vi "Grabber.vi"() -> ()   [LabVIEW 2013]
uses:
  <vilib>/userdefined/High Color/IMAQdx.ctl
  <vilib>/vision/Image Controls.llb/IMAQ Image.ctl
  CameraLan.lvclass
  <instrlib>/niHWS/nihws.llb/niHWS Open File Permissions ID.ctl
  <vilib>/Analysis/baseanly.llb/Mean (DBL).vi
  <vilib>/DAQmx/write.llb/DAQmx Write (Digital Bool 1Line 1Point).vi
  <vilib>/DAQmx/read.llb/DAQmx Read (Digital Bool 1Line 1Point).vi
  <instrlib>/niHWS/nihws.llb/niHWS Write Analog WDT.vi
  <instrlib>/niHWS/nihws.llb/niHWS Write Analog DBL.vi
  <vilib>/DAQmx/miscellaneous.llb/DAQmx Fill In Error Info.vi
  <vilib>/vision/NI_Vision_Development_Module.lvlib
  <vilib>/Analysis/NI_AALBase.lvlib
  <vilib>/ptbypt/NI_PtbyPt.lvlib
panel:
  out "ElectricalTrace 2":dbl format="%0.2f"
  in  "Threshold":dbl=4.0 format="%#_13g"
  in  "Sample":bool
  in  "Method":u16(ring) items=["Electrical/Optical"=3, "Electrical"=2, "Optical"=1, "Electrical+Optical"=0]
  out "Lick":bool
  out "Resistance \n      Lick":bool
  out "mean":dbl format="%0.2f"
  out "std":dbl format="%0.2f"
  out "ElectricalTrace":dynamicdata(graph)
  in  "Threshold":dbl=0.8 format="%#_13g"
  out "Crop Error":errorcluster
  out "Crop":T1(plugin-control)
  out "OpticalTrace":dbl(graph)
  out "Camera\n    Lick":bool
  in  "Lick \nDetection":bool
  in  "Display":bool
  out "Image Out":T1
  in  "Default path":string="F:\\Camera\\"
  out "Juice":bool
  in  "ExposureTime":dbl(slide)=1000.0 caption="Gain" scale=0.0..16466.666666666668
  in  "Magnify":bool
  in  "stop":bool
  in  "Compressor":string(combo)="DV Video Encoder"
  in  "quality":i32=-1
  in  "Rec":bool
  in  "Path":path
  in  "Gain":dbl(slide)=2.9811320754716983 min=1.0 max=16466.666666666668 scale=1.0..4.0
  out "acquired FPS":dbl
  out "Image":T1(plugin-control)
  in  "Session In":T2="S1028197"
  in  "Fps":i32=60
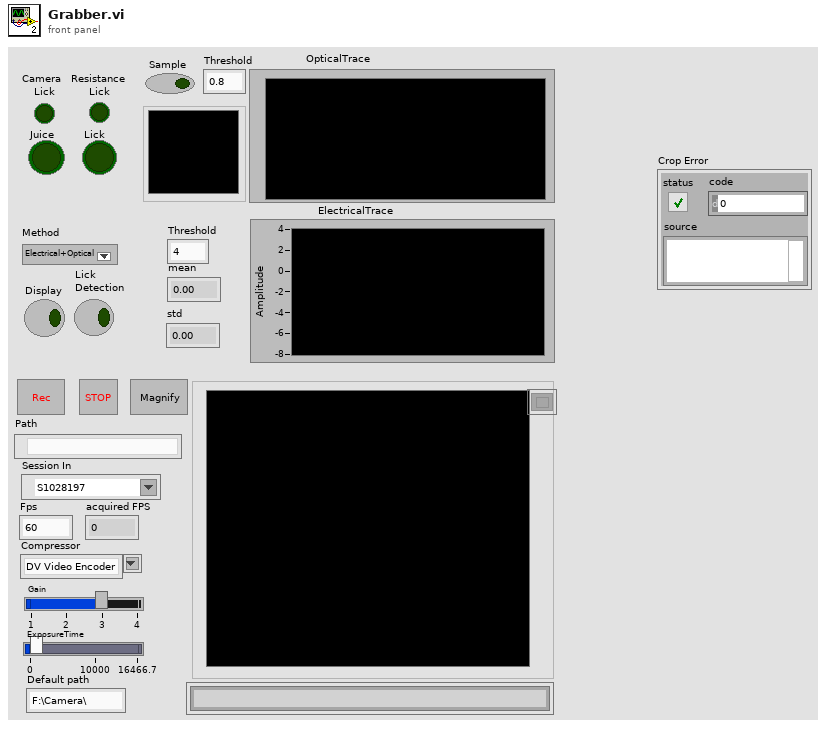
[diagram p1: front panel]
types:
  T1 = typedef "IMAQ Image.ctl" = refnum<image>
  T2 = typedef "IMAQdx.ctl" = refnum<k21>
  T3 = enum32{"Invalid", "Standard", "Closed", "Hidden", "Minimized", "Maximized"}
  T4 = typedef "niHWS Open File Permissions ID.ctl" = enum32{"Read Only", "Read/Write Existing", "Read/Write/Create New", "Read/Write/Create New Always"}
  T5 = typedef "AviRefnum.ctl" = refnum<k1>
  T6 = cluster{"Global Rectangle":i32[], "Contours":cluster{"Contour Type":u32, "ROI Type":u32, "Points":i32[]}[]}
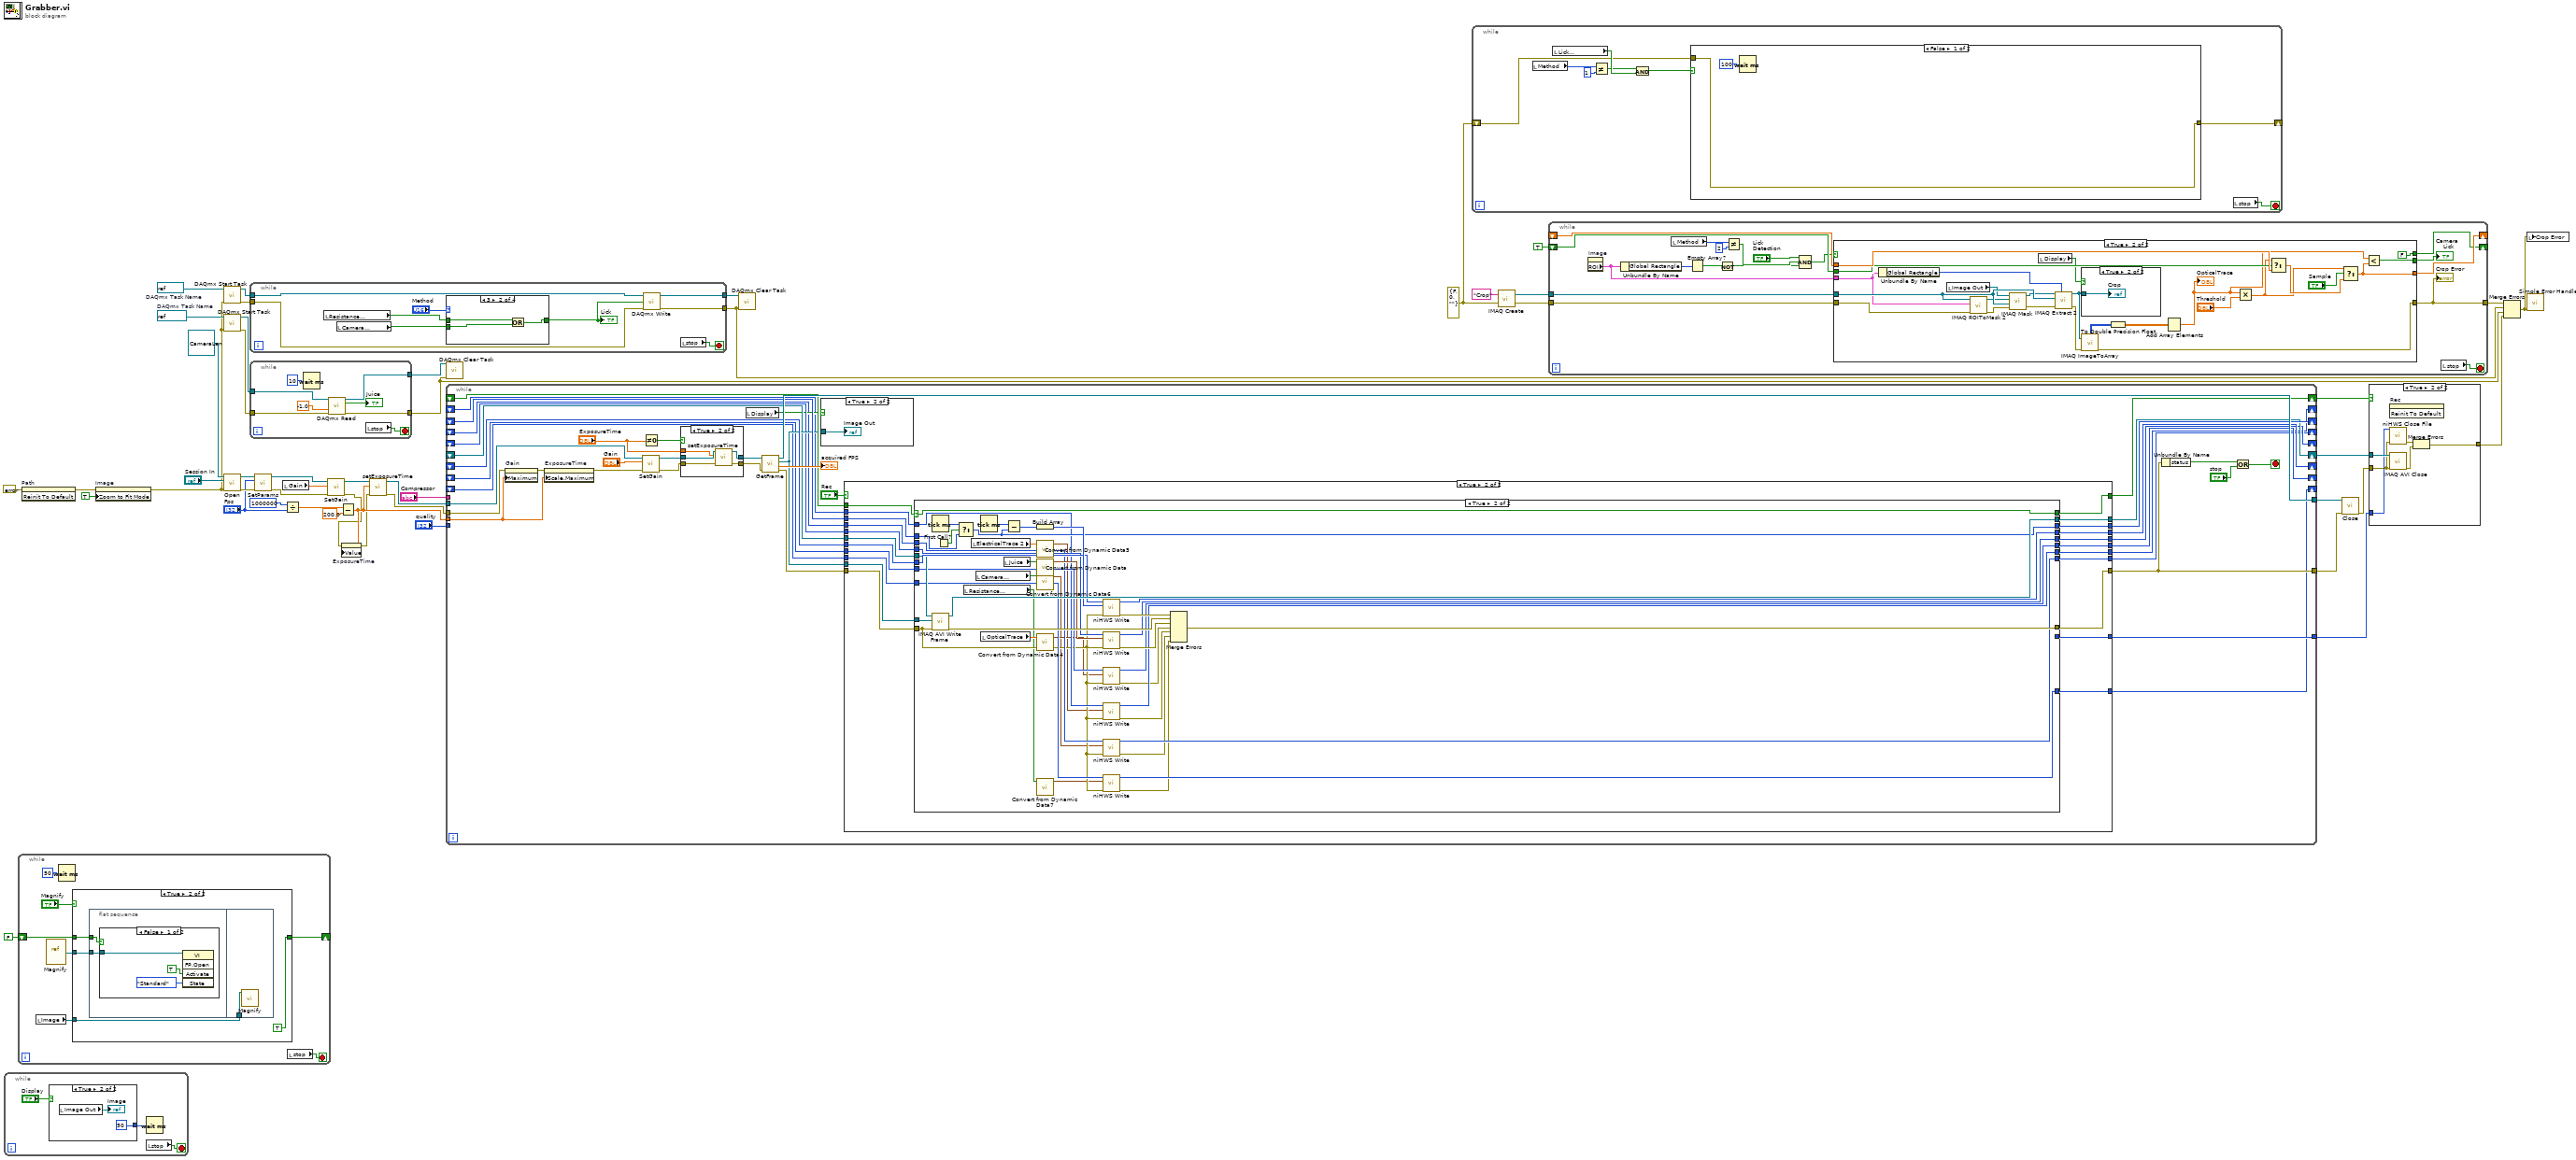
[diagram p0: block diagram]
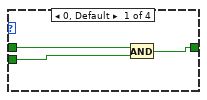
[diagram p2: hidden frame]
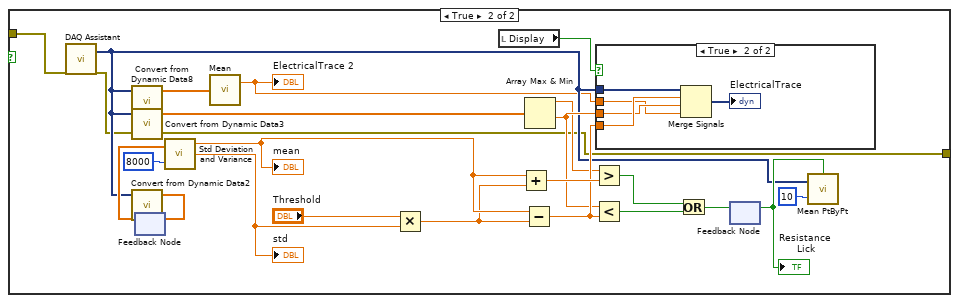
[diagram p5: hidden frame]
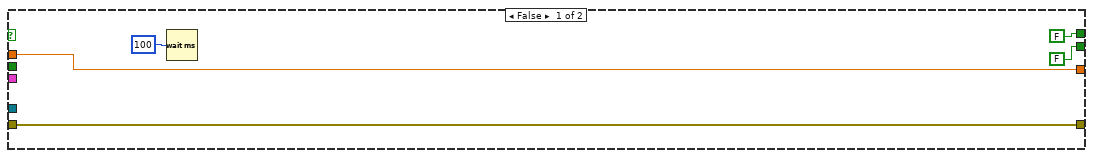
[diagram p7: hidden frame]
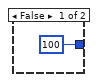
[diagram p9: hidden frame]
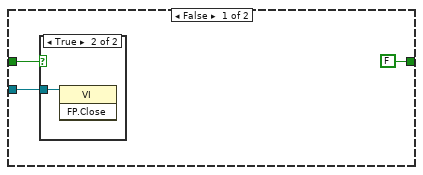
[diagram p10: hidden frame]
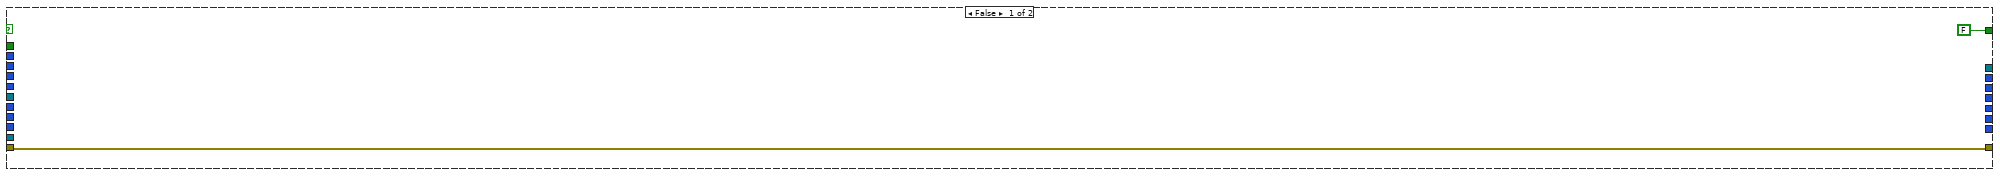
[diagram p16: hidden frame]
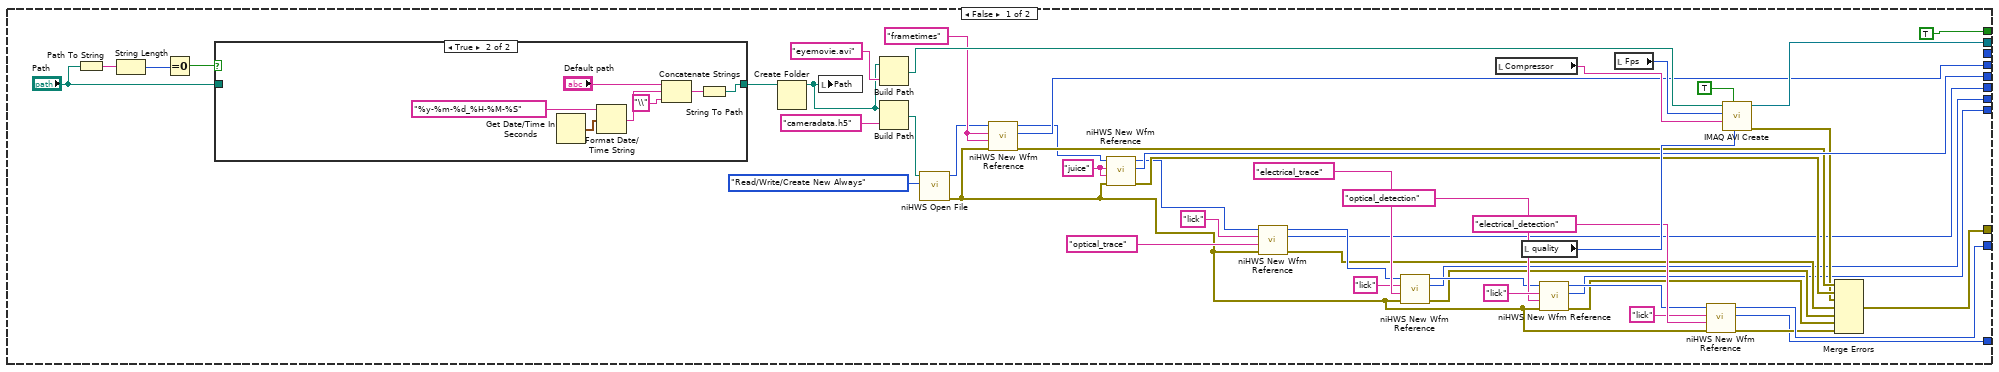
[diagram p17: hidden frame]
diagram:
  w21 = refnum<k21> "Lick"  # DAQmx Task Name
  w15 = errorcluster {"status"=FALSE, "code"=0, "source"=""} ("error in (no error)")
  w32 = refnum<k21> "Juice"  # DAQmx Task Name
  n1 = while {
    stop <- w51 stop-if-true
    n2 = case shown="True" "Display" {
      tunnel: [u32 100 ("milliseconds to wait") u32 50 ("milliseconds to wait")] -> w50
      frame False {
      }
      frame True {
        n3 = local read "Image Out"() -> (→"Image":T1)
      }
    }
    n4 = Wait (ms)(milliseconds to wait=w50) -> ()  [unwired: 1 out]
    n5 = local read "stop"() -> (w51:bool)
  }
  n6 = while {
    shift-right: [w59] -> _
    shift-left: FALSE -> [w58]
    stop <- w56 stop-if-true
    n7 = local read "Image"() -> (w55:T1)
    n8 = vi-ref "Magnify.vi"() -> (w61:refnum<vi>)
    n9 = Wait (ms)(milliseconds to wait=u32 50) -> ()  [unwired: 1 out]
    n10 = case shown="True" "Magnify" {
      tunnel: w61 -> [w64 w69]
      tunnel: [FALSE TRUE] -> w59
      tunnel: w58 -> [w63 w67]
      tunnel: w55 -> [_ w66]
      frame False {
        n11 = case shown="True" w63 {
          tunnel: w64 -> [_ w65]
          frame False {
          }
          frame True {
            n12 = invoke class="VI" method="FP.Close"(reference=w65) -> ()  [unwired: 2 in, 3 out]
          }
        }
      }
      frame True {
        n13 = flat-sequence {
          tunnel: w69 -> [w71]
          tunnel: w67 -> [w70]
          tunnel: w66 -> [w75]
          frame #0 {
            n14 = case shown="False" w70 {
              tunnel: w71 -> [w73 _]
              frame False {
                n15 = invoke class="VI" method="FP.Open"(reference=w73, "Activate"=TRUE ("Wait Until Done"), "State"=T3."Standard") -> ()  [unwired: 2 in, 5 out]
              }
              frame True {
              }
            }
          }
          frame #1 {
            n16 = call "Magnify.vi"("Camera 2"=w75) -> ()  [unwired: 11 in]
          }
        }
      }
    }
    n17 = local read "stop"() -> (w56:bool)
  }
  n18 = invoke on="Path" class="Path" method="Reinit To Default"(error in=errorcluster {"status"=FALSE, "code"=0, "source"=""} ("error in (no error)")) -> (error out=w22:errorcluster)  [unwired: 2 in, 2 out]
  n19 = property on="Image" class="ImageControl"(error in=w22, "Zoom to Fit Mode"=TRUE) -> (error out=w17:errorcluster)  [unwired: 1 in, 1 out]
  n20 = call <vilib>:"DAQmx Start Task.vi"("task/channels in"=w21, "error in"=w17) -> ("task out"=w19:refnum<k21>, "error out"=w18:errorcluster)  [unwired: 12 in]
  n21 = call <vilib>:"DAQmx Start Task.vi"("task/channels in"=w32, "error in"=w17) -> ("task out"=w33:refnum<k21>, "error out"=w31:errorcluster)  [unwired: 12 in]
  n22 = call-dynamic "Open.vi"("error in (no error)"=w17, "Session In"="Session In", "CameraLan in"=refnum<class "CameraLan.lvclass"> refnum) -> ("error out"=w47:errorcluster, "CameraLan out"=w46:refnum<class "CameraLan.lvclass">)  [unwired: 7 in]
  n23 = while {
    tunnel: [w83] -> w20
    tunnel: [w82] -> w13
    tunnel: w19 -> [w81]
    tunnel: w18 -> [w80]
    stop <- w84 stop-if-true
    n24 = local read "Resistance \n      Lick"() -> (w78:bool)
    n25 = local read "Camera\n    Lick"() -> (w77:bool)
    n26 = case shown="3" "Method" {
      tunnel: w78 -> [w87 w90 _ w92]
      tunnel: w77 -> [w86 w89 w91 _]
      tunnel: [w85 w88 w91 w92] -> w76
      frame 0, Default {
        n27 = And(x=w87, y=w86) -> (x .and. y?=w85:bool)
      }
      frame 3 {
        n28 = Or(x=w90, y=w89) -> (x .or. y?=w88:bool)
      }
      frame 1 {
      }
      frame 2 {
      }
    }
    "Lick" <- w76
    n29 = call-poly <vilib>:"DAQmx Write.vi"("task/channels in"=w81, "data"=w76, "error in"=w80) -> ("task out"=w83:refnum<k21>, "error out"=w82:errorcluster)  [unwired: 10 in, 1 out]
    n30 = local read "stop"() -> (w84:bool)
  }
  n31 = while {
    tunnel: w33 -> [w97]
    tunnel: w31 -> [w96]
    tunnel: [w95] -> w30
    tunnel: [w94] -> w12
    stop <- w100 stop-if-true
    n32 = Wait (ms)(milliseconds to wait=u32 10) -> ()  [unwired: 1 out]
    n33 = call-poly <vilib>:"DAQmx Read.vi"("task/channels in"=w97, "timeout"=-1.0, "error in"=w96) -> ("task out"=w95:refnum<k21>, "data"=→"Juice":bool, "error out"=w94:errorcluster)  [unwired: 10 in]
    n34 = local read "stop"() -> (w100:bool)
  }
  n35 = call-dynamic "SetParams.vi"("error in (no error)"=w47, "Fps"="Fps", "CameraLan in"=w46) -> ("error out"=w6:errorcluster, "CameraLan out"=w8:refnum<class "CameraLan.lvclass">)  [unwired: 7 in]
  n36 = local read "Gain"() -> (w4:dbl)
  n37 = Divide(x=1000000, y="Fps") -> (x/y=w37:dbl)
  n38 = call-dynamic "SetGain.vi"("error in (no error)"=w6, "Gain"=w4, "CameraLan in"=w8) -> ("error out"=w2:errorcluster, "CameraLan out"=w9:refnum<class "CameraLan.lvclass">)  [unwired: 7 in]
  n39 = Subtract(x=w37, y=200.0) -> (x-y=w3:dbl)
  n40 = property on="ExposureTime" class="Slide (strict)"(error in=w2, "Value"=w3) -> (error out=w1:errorcluster)  [unwired: 1 in, 1 out]
  n41 = call-dynamic "setExposureTime.vi"("error in (no error)"=w1, "ExposureTime"=w3, "CameraLan in"=w9) -> ("error out"=w5:errorcluster, "CameraLan out"=w7:refnum<class "CameraLan.lvclass">)  [unwired: 7 in]
  n42 = call <vilib>:"DAQmx Clear Task.vi"("task in"=w30, "error in"=w12) -> ()  [unwired: 13 in, 1 out]
  n43 = while {
    tunnel: [w141] -> w48
    tunnel: w7 -> [w140]
    tunnel: w5 -> [w117]
    tunnel: "Compressor" -> [_]
    tunnel: "quality" -> [_]
    shift-right: [w136] -> w41
    shift-left: _ -> [w135]
    shift-right: [w134] -> _
    shift-left: _ -> [w133]
    shift-right: [w132] -> _
    shift-left: _ -> [w131]
    tunnel: [w129] -> w39
    tunnel: [w112] -> w29
    shift-right: [w130] -> w40
    shift-left: _ -> [w127]
    tunnel: w3 -> [w120]
    shift-right: [w119] -> _
    shift-left: _ -> [w110]
    shift-right: [w108] -> _
    shift-left: _ -> [w104]
    shift-right: [w107] -> _
    shift-left: _ -> [w103]
    shift-right: [w106] -> _
    shift-left: _ -> [w102]
    shift-right: [w105] -> _
    shift-left: _ -> [w101]
    stop <- w113 stop-if-true
    n44 = property on="Gain" class="Slide (strict)"(error in=w117, "Maximum"=w120) -> (error out=w118:errorcluster)  [unwired: 1 in, 1 out]
    n45 = property on="ExposureTime" class="Slide (strict)"(error in=w118, "Scale.Maximum"=w120) -> (error out=w116:errorcluster)  [unwired: 1 in, 1 out]
    n46 = call-dynamic "SetGain.vi"("error in (no error)"=w116, "Gain"="Gain", "CameraLan in"=w140) -> ("error out"=w124:errorcluster, "CameraLan out"=w126:refnum<class "CameraLan.lvclass">)  [unwired: 7 in]
    n47 = Not Equal To 0?(x="ExposureTime") -> (x != 0?=w121:bool)
    n48 = case shown="True" w121 {
      tunnel: w126 -> [w144 w149]
      tunnel: [w144 w148] -> w125
      tunnel: w124 -> [w143 w147]
      tunnel: [w143 w146] -> w123
      tunnel: "ExposureTime" -> [_ w145]
      frame False {
      }
      frame True {
        n49 = call-dynamic "setExposureTime.vi"("error in (no error)"=w147, "ExposureTime"=w145, "CameraLan in"=w149) -> ("error out"=w146:errorcluster, "CameraLan out"=w148:refnum<class "CameraLan.lvclass">)  [unwired: 7 in]
      }
    }
    n50 = local read "Display"() -> (w109:bool)
    n51 = call-dynamic "GetFrame.vi"("error in (no error)"=w123, "CameraLan in"=w125) -> ("error out"=w115:errorcluster, "acquired FPS"=→"acquired FPS":dbl, "Image Out"=w128:T1, "CameraLan out"=w141:refnum<class "CameraLan.lvclass">)  [unwired: 5 in, 1 out]
    n52 = case shown="True" w109 {
      tunnel: w128 -> [_ w142]
      frame False {
      }
      frame True {
        "Image Out" <- w142
      }
    }
    n53 = case shown="True" "Rec" {
      tunnel: [_ w172] -> w130
      tunnel: [FALSE w173] -> w136
      tunnel: [_ w171] -> w132
      tunnel: w135 -> [_ w170]
      tunnel: [_ w169] -> w134
      tunnel: w133 -> [_ w168]
      tunnel: w131 -> [_ w167]
      tunnel: [_ w166] -> w129
      tunnel: [w150 w165] -> w112
      tunnel: w128 -> [_ w164]
      tunnel: w127 -> [_ w163]
      tunnel: [_ w162] -> w119
      tunnel: w115 -> [w150 w161]
      tunnel: w110 -> [_ w160]
      tunnel: [_ w159] -> w108
      tunnel: [_ w158] -> w107
      tunnel: [_ w157] -> w106
      tunnel: [_ w156] -> w105
      tunnel: w104 -> [_ w155]
      tunnel: w103 -> [_ w154]
      tunnel: w102 -> [_ w153]
      tunnel: w101 -> [_ w152]
      frame False {
      }
      frame True {
        n54 = case shown="True" w170 {
          selector: w170 -> [_ w272]
          tunnel: [TRUE w272] -> w173
          tunnel: [w219 w271] -> w172
          tunnel: [w204 w265] -> w171
          tunnel: [_ w260] -> w169
          tunnel: w168 -> [_ w268]
          tunnel: w167 -> [_ w266]
          tunnel: [w183 _] -> w166
          tunnel: [w198 w257] -> w165
          tunnel: w164 -> [_ w263]
          tunnel: w163 -> [_ w262]
          tunnel: [w201 w255] -> w162
          tunnel: w161 -> [_ w239]
          tunnel: w160 -> [_ w254]
          tunnel: [w177 w251] -> w159
          tunnel: [w176 w250] -> w158
          tunnel: [w175 w249] -> w157
          tunnel: [w174 w248] -> w156
          tunnel: w155 -> [_ w243]
          tunnel: w154 -> [_ w242]
          tunnel: w153 -> [_ w241]
          tunnel: w152 -> [_ w240]
          frame False {
            w203 = "juice" ("group name (empty)")
            w208 = "frametimes" ("group name (empty)")
            n55 = Path To String(path="Path") -> (string=w220:string)
            n56 = String Length(string=w220) -> (length=w221:i32)
            n57 = Equal To 0?(x=w221) -> (x = 0?=w212:bool)
            n58 = case shown="True" w212 {
              tunnel: [w223 w224] -> w210
              tunnel: "Path" -> [w223 _]
              frame False {
              }
              frame True {
                n59 = Get Date/Time In Seconds() -> (seconds since 1Jan1904=w230:timestamp)
                n60 = Format Date/Time String(time format string (%c)="%y-%m-%d_%H-%M-%S", seconds (now)=w230) -> (date/time string=w227:string)  [unwired: 1 in]
                n61 = Concatenate Strings("Default path", w227, "\\" ("string")) -> (w225:string)
                n62 = String To Path(string=w225) -> (path=w224:path)
              }
            }
            n63 = Create Folder(path (use dialog)=w210) -> (created path=w209:path)  [unwired: 2 in, 2 out]
            n64 = local write "Path"(w209) -> ()
            n65 = Build Path(base path=w209, name or relative path="eyemovie.avi" ("search string")) -> (appended path=w215:path)
            n66 = Build Path(base path=w209, name or relative path="cameradata.h5" ("search string")) -> (appended path=w213:path)
            n67 = call <instrlib>:"niHWS Open File.vi"("permissions (0:read only)"=niHWS_Open_File_Permissions_ID."Read/Write/Create New Always", "file path"=w213) -> ("error out"=w182:errorcluster, "file handle"=w202:u32)  [unwired: 8 in]
            n68 = call <instrlib>:"niHWS New Wfm Reference.vi"("error in (no error)"=w182, "waveform name (empty)"=w208, "group name (empty)"=w208, "file handle in"=w202) -> ("error out"=w199:errorcluster, "waveform reference"=w204:u32, "file handle out"=w196:u32)  [unwired: 5 in]
            n69 = call <instrlib>:"niHWS New Wfm Reference.vi"("error in (no error)"=w182, "waveform name (empty)"=w203, "group name (empty)"=w203, "file handle in"=w196) -> ("error out"=w200:errorcluster, "waveform reference"=w201:u32, "file handle out"=w195:u32)  [unwired: 5 in]
            n70 = call <instrlib>:"niHWS New Wfm Reference.vi"("error in (no error)"=w182, "waveform name (empty)"="optical_trace", "group name (empty)"="lick", "file handle in"=w195) -> ("error out"=w181:errorcluster, "waveform reference"=w177:u32, "file handle out"=w186:u32)  [unwired: 5 in]
            n71 = call <instrlib>:"niHWS New Wfm Reference.vi"("error in (no error)"=w182, "waveform name (empty)"="electrical_trace", "group name (empty)"="lick", "file handle in"=w186) -> ("error out"=w180:errorcluster, "waveform reference"=w176:u32, "file handle out"=w185:u32)  [unwired: 5 in]
            n72 = local read "Compressor"() -> (w206:string)
            n73 = local read "quality"() -> (w205:i32)
            n74 = call <instrlib>:"niHWS New Wfm Reference.vi"("error in (no error)"=w182, "waveform name (empty)"="optical_detection", "group name (empty)"="lick", "file handle in"=w185) -> ("error out"=w179:errorcluster, "waveform reference"=w175:u32, "file handle out"=w184:u32)  [unwired: 5 in]
            n75 = local read "Fps"() -> (w207:i32)
            n76 = call <instrlib>:"niHWS New Wfm Reference.vi"("error in (no error)"=w182, "waveform name (empty)"="electrical_detection", "group name (empty)"="lick", "file handle in"=w184) -> ("error out"=w178:errorcluster, "waveform reference"=w174:u32, "file handle out"=w183:u32)  [unwired: 5 in]
            n77 = call "IMAQ AVI Create"("quality"=w205, "Has Data"=TRUE, "Compression Filter"=w206, "Frames Per Second"=w207, "AVI Path"=w215) -> ("error out"=w197:errorcluster, "Avi Refnum"=w219:T5)  [unwired: 2 in, 3 out]
            n78 = Merge Errors(w199, w200, w197, w181, w180, w179, w178) -> (w198:errorcluster)
          }
          frame True {
            n79 = Tick Count (ms)() -> (millisecond timer value=w269:u32)
            n80 = call "IMAQ AVI Write Frame"("error in (no error)"=w239, "Image"=w263, "Avi Refnum"=w262) -> ("error out"=w258:errorcluster, "Avi Refnum (duplicate)"=w271:T5)  [unwired: 7 in]
            n81 = First Call?() -> (First Call?: T/F=w270:bool)
            n82 = Select(t=w269, s=w270, f=w268) -> (s? t:f=w260:u32)
            n83 = local read "Resistance \n      Lick"() -> (w231:bool)
            n84 = local read "ElectricalTrace 2"() -> (w233:dbl)
            n85 = local read "Camera\n    Lick"() -> (w232:bool)
            n86 = Tick Count (ms)() -> (millisecond timer value=w261:u32)
            n87 = local read "OpticalTrace"() -> (w237:dbl)
            n88 = local read "Juice"() -> (w253:bool)
            n89 = Subtract(x=w261, y=w260) -> (x-y=w264:u32)
            n90 = Build Array(w264) -> (w267:u32[])
            n91 = call "Convert from Dynamic Data5"("Dynamic Data Type"=w233) -> ("Waveform"=w236:waveform(dbl))  [unwired: 3 in]
            n92 = call "Convert from Dynamic Data"("Dynamic Data Type"=w253) -> ("Waveform"=w252:waveform(dbl))  [unwired: 3 in]
            n93 = call "Convert from Dynamic Data6"("Dynamic Data Type"=w232) -> ("Waveform"=w235:waveform(dbl))  [unwired: 3 in]
            n94 = call "Convert from Dynamic Data4"("Dynamic Data Type"=w237) -> ("Waveform"=w238:waveform(dbl))  [unwired: 3 in]
            n95 = call "Convert from Dynamic Data7"("Dynamic Data Type"=w231) -> ("Waveform"=w234:waveform(dbl))  [unwired: 3 in]
            n96 = call-poly <instrlib>:"niHWS Write.vi"("error in (no error)"=w239, "data"=w267, "waveform reference in"=w266) -> ("error out"=w259:errorcluster, "waveform reference out"=w265:u32)  [unwired: 7 in]
            n97 = call-poly <instrlib>:"niHWS Write.vi"("error in (no error)"=w239, "analog waveform"=w252, "waveform reference in"=w254) -> ("error out"=w256:errorcluster, "waveform reference out"=w255:u32)  [unwired: 7 in]
            n98 = call-poly <instrlib>:"niHWS Write.vi"("error in (no error)"=w239, "analog waveform"=w238, "waveform reference in"=w243) -> ("error out"=w247:errorcluster, "waveform reference out"=w251:u32)  [unwired: 7 in]
            n99 = call-poly <instrlib>:"niHWS Write.vi"("error in (no error)"=w239, "analog waveform"=w236, "waveform reference in"=w242) -> ("error out"=w246:errorcluster, "waveform reference out"=w250:u32)  [unwired: 7 in]
            n100 = call-poly <instrlib>:"niHWS Write.vi"("error in (no error)"=w239, "analog waveform"=w235, "waveform reference in"=w241) -> ("error out"=w245:errorcluster, "waveform reference out"=w249:u32)  [unwired: 7 in]
            n101 = call-poly <instrlib>:"niHWS Write.vi"("error in (no error)"=w239, "analog waveform"=w234, "waveform reference in"=w240) -> ("error out"=w244:errorcluster, "waveform reference out"=w248:u32)  [unwired: 7 in]
            n102 = Merge Errors(w259, w258, w256, w247, w246, w245, w244) -> (w257:errorcluster)
          }
        }
      }
    }
    n103 = Unbundle By Name(w112) -> ("status"=w111:bool)
    n104 = Or(x=w111, y="stop") -> (x .or. y?=w113:bool)
  }
  n105 = call <vilib>:"DAQmx Clear Task.vi"("task in"=w20, "error in"=w13) -> ()  [unwired: 13 in, 1 out]
  n106 = while {
    shift-right: [w274] -> _
    shift-left: w15 -> [w273]
    stop <- w280 stop-if-true
    n107 = local read "Method"() -> (w278:u16)
    n108 = local read "Lick \nDetection"() -> (w277:bool)
    n109 = Not Equal?(x=w278, y=u16 1) -> (x != y?=w276:bool)
    n110 = And(x=w276, y=w277) -> (x .and. y?=w275:bool)
    n111 = case shown="False" w275 {
      tunnel: [w281 w284] -> w274
      tunnel: w273 -> [w281 w283]
      frame False {
        n112 = Wait (ms)(milliseconds to wait=u32 100) -> ()  [unwired: 1 out]
      }
      frame True {
        n113 = call "DAQ Assistant"("error in"=w283) -> ("data"=w287:dynamicdata, "error out"=w284:errorcluster)  [unwired: 15 in, 2 out]
        n114 = call "Convert from Dynamic Data8"("Dynamic Data Type"=w287) -> ("Array"=w286:dbl[])  [unwired: 3 in]
        n115 = call "Convert from Dynamic Data3"("Dynamic Data Type"=w287) -> ("Array"=w290:dbl[])  [unwired: 3 in]
        n116 = call "Convert from Dynamic Data2"("Dynamic Data Type"=w287) -> ("Array"=w292:dbl[])  [unwired: 3 in]
        n117 = feedback-in #1(w292) -> ()
        n118 = feedback #1() -> (w291:dbl[])  [unwired: 1 in]
        n119 = call <vilib>:"Std Deviation and Variance.vi"("X"=w291, "Weighting (Sample)"=8000 ("sample length")) -> ("mean"=w301:dbl, "standard deviation"=w303:dbl)  [unwired: 1 out]
        "mean" <- w301
        "std" <- w303
        n120 = call-poly <vilib>:"Mean.vi"("X"=w286) -> ("mean"=w285:dbl)  [unwired: 1 out]
        "ElectricalTrace 2" <- w285
        n121 = Multiply(x="Threshold", y=w303) -> (x*y=w300:dbl)
        n122 = local read "Display"() -> (w295:bool)
        n123 = Add(x=w301, y=w300) -> (x+y=w302:dbl)
        n124 = Subtract(x=w301, y=w300) -> (x-y=w293:dbl)
        n125 = Array Max & Min(array=w290) -> (max value=w288:dbl, min value=w289:dbl)  [unwired: 2 out]
        n126 = Greater?(x=w288, y=w302) -> (0:w299:bool)
        n127 = Less?(x=w289, y=w293) -> (x < y?=w298:bool)
        n128 = case shown="True" w295 {
          tunnel: w287 -> [_ w310]
          tunnel: w293 -> [_ w308]
          tunnel: w289 -> [_ w307]
          tunnel: w285 -> [_ w306]
          frame False {
          }
          frame True {
            n129 = Merge Signals(w310, w308, w307, w306) -> (→"ElectricalTrace":dynamicdata)
          }
        }
        n130 = Or(x=w299, y=w298) -> (x .or. y?=w297:bool)
        n131 = feedback #2() -> (w296:bool)  [unwired: 1 in]
        "Resistance \n      Lick" <- w296
        n132 = feedback-in #2(w297) -> ()
        n133 = call <vilib>:"Mean PtByPt.vi"("x"=w287, "sample length"=10, "initialize"=w296) -> ()  [unwired: 1 in, 2 out]
      }
    }
    n134 = local read "stop"() -> (w280:bool)
  }
  n135 = call "IMAQ Create"("Image Name"="Crop", "error in (no error)"=w15) -> ("New Image"=w26:T1, "error out"=w25:errorcluster)  [unwired: 3 in]
  n136 = while {
    shift-right: [w327] -> _
    shift-left: _ -> [w326]
    shift-right: [w325] -> _
    shift-left: TRUE -> [w324]
    tunnel: [w323] -> w14
    tunnel: w25 -> [w322]
    tunnel: w26 -> [w321]
    stop <- w328 stop-if-true
    n137 = property on="Image" class="ImageControl"() -> ("ROI"=w318:T6)  [unwired: 2 in, 2 out]
    n138 = Unbundle By Name(w318) -> ("Global Rectangle"=w317:i32[])
    n139 = local read "Method"() -> (w320:u16)
    n140 = Empty Array?(array=w317) -> (empty?=w316:bool)
    n141 = Not(x=w316) -> (.not. x?=w313:bool)
    n142 = Not Equal?(x=w320, y=u16 2) -> (x != y?=w314:bool)
    n143 = Compound Arithmetic op=AND("Lick \nDetection", w314, w313) -> (w312:bool)
    n144 = case shown="True" w312 {
      tunnel: w318 -> [_ w352]
      tunnel: [w331 w336] -> w327
      tunnel: w326 -> [w331 w358]
      tunnel: [FALSE FALSE] -> w325
      tunnel: w324 -> [_ w356]
      tunnel: [w332 w355] -> w323
      tunnel: w322 -> [w332 w354]
      tunnel: w321 -> [_ w353]
      tunnel: [FALSE w334] -> w319
      frame False {
        n145 = Wait (ms)(milliseconds to wait=u32 100) -> ()  [unwired: 1 out]
      }
      frame True {
        n146 = Unbundle By Name(w352) -> ("Global Rectangle"=w351:i32[])
        n147 = local read "Image Out"() -> (w343:T1)
        n148 = call "IMAQ ROIToMask 2"("error in (no error)"=w354, "ROI Descriptor"=w352, "Image"=w353) -> ("error out"=w342:errorcluster, "Image Out"=w344:T1)  [unwired: 6 in, 1 out]
        n149 = call "IMAQ Mask"("error in (no error)"=w342, "Image Dst"=w353, "Image Mask"=w344, "Image Src"=w343) -> ("error out"=w341:errorcluster, "Image Dst Out"=w350:T1)  [unwired: 1 in]
        n150 = local read "Display"() -> (w339:bool)
        n151 = call "IMAQ Extract 2"("Optional Rectangle"=w351, "error in (no error)"=w341, "Image Dst"=w353, "Image Src"=w350) -> ("error out"=w340:errorcluster, "Image Dst Out"=w349:T1)  [unwired: 6 in]
        n152 = case shown="True" w339 {
          tunnel: w349 -> [_ w359]
          frame False {
          }
          frame True {
            "Crop" <- w359
          }
        }
        n153 = call "IMAQ ImageToArray"("error in (no error)"=w340, "Image"=w349) -> ("error out"=w355:errorcluster, "Image Pixels (U8)"=w347:u8[][])  [unwired: 2 in, 3 out]
        n154 = To Double Precision Float(number=w347) -> (double precision float=w348:dbl[][])
        n155 = Add Array Elements(numeric array=w348) -> (sum=w345:dbl)
        "OpticalTrace" <- w345
        n156 = Multiply(x=w345, y="Threshold") -> (x*y=w337:dbl)
        n157 = Select(t=w337, s=w356, f=w358) -> (s? t:f=w338:dbl)
        n158 = Select(t=w337, s="Sample", f=w338) -> (s? t:f=w336:dbl)
        n159 = Less?(x=w345, y=w336) -> (x < y?=w334:bool)
      }
    }
    "Crop Error" <- w323
    "Camera\n    Lick" <- w319
    n160 = local read "stop"() -> (w328:bool)
  }
  n161 = call-dynamic "Close.vi"("error in (no error)"=w29, "CameraLan in"=w48) -> ("error out"=w28:errorcluster)  [unwired: 9 in]
  n162 = case shown="True" w41 {
    tunnel: w40 -> [_ w366]
    tunnel: w39 -> [_ w365]
    tunnel: w28 -> [w360 w364]
    tunnel: [w360 w361] -> w11
    frame False {
    }
    frame True {
      n163 = call <instrlib>:"niHWS Close File.vi"("error in (no error)"=w364, "file handle"=w365) -> ("error out"=w363:errorcluster)  [unwired: 9 in]
      n164 = call "IMAQ AVI Close"("error in (no error)"=w364, "Avi Refnum"=w366) -> ("error out"=w362:errorcluster)  [unwired: 9 in]
      n165 = invoke on="Rec" class="Bool (strict)" method="Reinit To Default"() -> ()  [unwired: 3 in, 3 out]
      n166 = Merge Errors(w363, w362) -> (w361:errorcluster)
    }
  }
  n167 = Merge Errors(w14, w13, w12, w11) -> (w10:errorcluster)
  n168 = local write "Crop Error"(w10) -> ()
  n169 = call <vilib>:"Simple Error Handler.vi"("error in (no error)"=w10) -> ()  [unwired: 4 in, 5 out]
